vi "Get CT Offsets.vi"(8 "Error In":errorcluster, 11 "Path":path) -> (0 "Error Out":errorcluster, 3 "CT Offsets":fxp<+,24,6>[](array[numeric]))   [LabVIEW 2013]
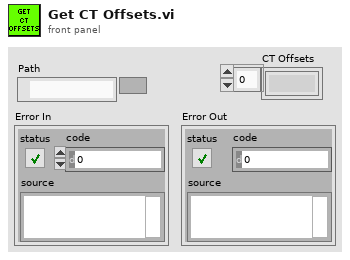
[diagram p1: front panel]
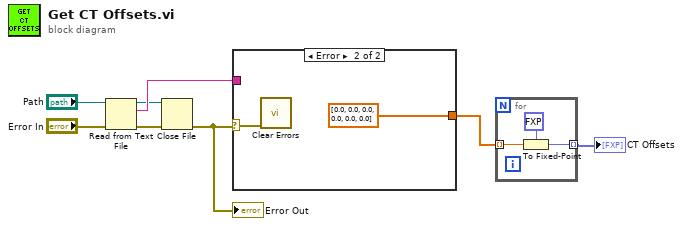
[diagram p0: block diagram]
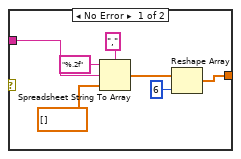
[diagram p2: hidden frame]
diagram:
  n1 = Read from Text File(file (use dialog)="Path", error in="Error In") -> (refnum out=w7:refnum<file>, text=w8:string, error out=w6:errorcluster)  [unwired: 2 in, 1 out]
  n2 = Close File(refnum=w7, error in=w6) -> (error out=w4:errorcluster)  [unwired: 1 out]
  "Error Out" <- w4
  n3 = case shown="Error" w4 {
    selector: w4 -> [_ w17]
    tunnel: w8 -> [w13 _]
    tunnel: [w9 dbl[] [0.0, 0.0, 0.0, 0.0, 0.0, 0.0]] -> w3
    frame No Error {
      n4 = Spreadsheet String To Array(delimiter (Tab)=",", format string="%.2f", spreadsheet string=w13, array type (2D Dbl)=dbl[] []) -> (array=w11:dbl[])
      n5 = Reshape Array(w11, 6 ("dimension size")) -> (w9:dbl[])
    }
    frame Error {
      n6 = call <vilib>:"Clear Errors.vi"("error in (no error)"=w17) -> ()  [unwired: 6 in, 1 out]
    }
  }
  n7 = for {
    tunnel: w3 -> [w20] mode=indexing
    tunnel: [w18] -> w2 mode=indexing
    n8 = To Fixed-Point(fixed-point type=fxp<+,24,6> 0.0 ("RMS"), number=w20) -> (fixed-point=w18:fxp<+,24,6>)
  }
  "CT Offsets" <- w2
